vi "LH_ReleaseList.vi"(3 "InputList":refnum<class "ListHead.lvclass">) -> ()   [LabVIEW 2014, in "ListHead.lvclass"]
uses:
  ListHead.lvclass
  ListHead.lvclass/ListHead.ctl
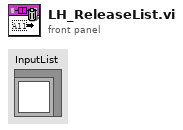
[diagram p1: front panel]
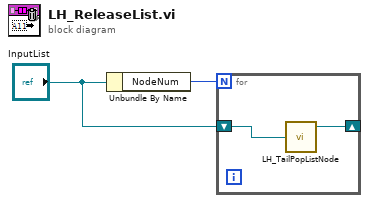
[diagram p0: block diagram]
diagram:
  n1 = Unbundle By Name("InputList") -> ("NodeNum"=w2:u32)
  n2 = for {
    N: w2 -> [_]
    shift-right: [w3] -> _
    shift-left: "InputList" -> [w4]
    n3 = call "LH_TailPopListNode.vi"("InputList"=w4) -> ("OutputList"=w3:refnum<class "ListHead.lvclass">)  [unwired: 2 out]
  }
